vi "GetBusClass.vi"(8 "ErrorArray In":errorcluster[](array[cluster]), 9 "arg":string, 10 "BusNumber":u8) -> (0 "ErrorArray Out":errorcluster[](array[cluster]), 3 "Framework.lvlib:Bus.lvclass":refnum<class "Bus.lvclass">)   [LabVIEW 2017, in "Bus_class.lvlib" / "Bus.lvclass"]
uses:
  Bus.lvclass
  <vilib>/Utility/error.llb/Error Cluster From Error Code.vi
  <vilib>/ErrorRing/Error Ring.xnode
  <userlib>/NIST/NISTErrorLib/NISTErrorLib.lvlib
  Framework.lvlib
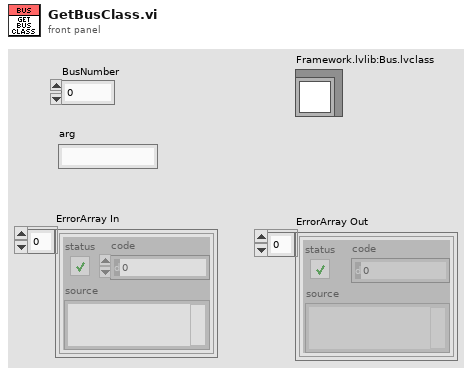
[diagram p1: front panel]
types:
  T1 = typedef "Framework.lvlib/clFrameworkData.ctl" = cluster{"EvtINIFilePaths":path[], "BusClassInstances":refnum<class "Bus.lvclass">[], "PmuImpairINIFilePaths":path[], "FlagImpairINIFilePaths":path[], "NetImpairINIFilePaths":path[], "OutputToFileINIFilePaths":path[], "AppINIFilePaths":path[], "AppModuleID":i32, "OutputToFileID":i32}
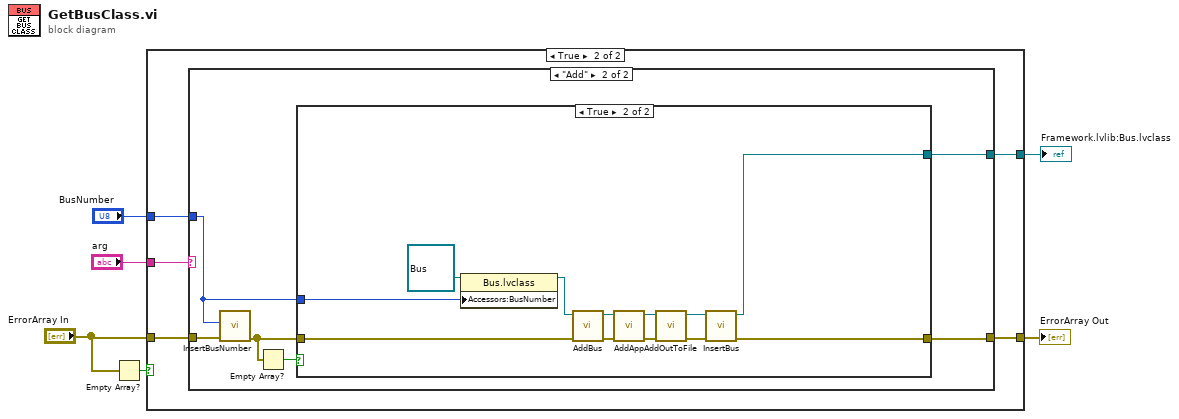
[diagram p0: block diagram]
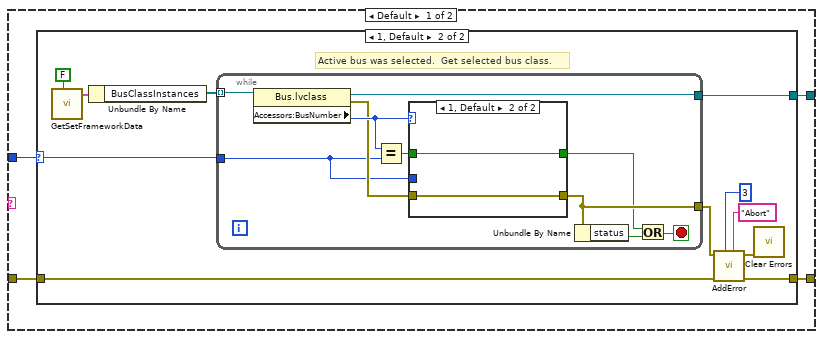
[diagram p3: hidden frame]
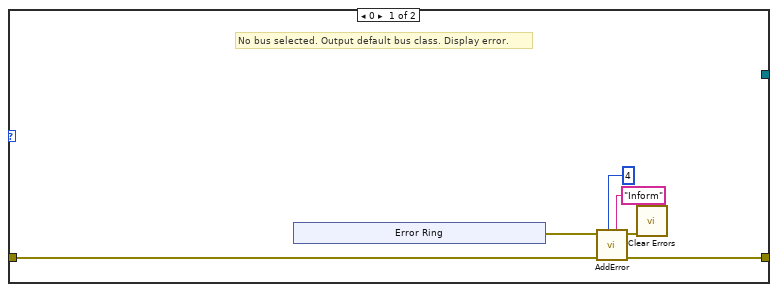
[diagram p4: hidden frame]
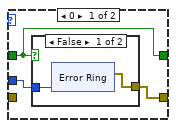
[diagram p5: hidden frame]
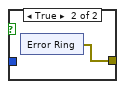
[diagram p6: hidden frame]
diagram:
  n1 = Empty Array?(array="ErrorArray In") -> (empty?=w2:bool)
  n2 = case shown="True" w2 {
    tunnel: "ErrorArray In" -> [w7 w11]
    tunnel: [w7 w12] -> w6
    tunnel: [_ w10] -> w5
    tunnel: "BusNumber" -> [_ w9]
    tunnel: "arg" -> [_ w8]
    frame False {
      # "External error.  Error array holds at least one error."
    }
    frame True {
      n3 = case shown="\"Add\"" w8 {
        tunnel: [w16 w70] -> w12
        tunnel: w11 -> [w15 w74]
        tunnel: [w14 w69] -> w10
        tunnel: w9 -> [w13 w71]
        frame Default {
          n4 = case shown="1, Default" w13 {
            selector: w13 -> [_ w32]
            tunnel: [w18 w38] -> w16
            tunnel: w15 -> [w19 w29]
            tunnel: [_ w31] -> w14
            frame 0 {
              # "No bus selected. Output default bus class. Display error."
              n5 = xnode "Error Ring"() -> ("error out"=w17:errorcluster)
              n6 = call <userlib>:"AddError.vi"("Severity"="Inform" ("String"), "Priority"=u8 4, "ErrorArray"=w19, "error in (no error)"=w17) -> ("ErrorArray"=w18:errorcluster[], "error out"=w22:errorcluster)  [unwired: 6 in]
              n7 = call <vilib>:"Clear Errors.vi"("error in (no error)"=w22) -> ()  [unwired: 5 in, 2 out]
            }
            frame 1, Default {
              # "Active bus was selected.  Get selected bus class."
              n8 = call "GetSetFrameworkData.vi"("Set (F)"=FALSE ("Set/Get")) -> ("clFrameworkData Out"=w33:T1)  [unwired: 10 in]
              n9 = Unbundle By Name(w33) -> ("BusClassInstances"=w30:refnum<class "Bus.lvclass">[])
              n10 = while {
                tunnel: w32 -> [w41]
                tunnel: [w48] -> w31
                tunnel: w30 -> [w47] mode=indexing
                tunnel: [w42] -> w28
                stop <- w45 stop-if-true
                n11 = property class="Bus.lvclass"(reference=w47) -> (reference out=w48:refnum<class "Bus.lvclass">, error out=w43:errorcluster, "Accessors:BusNumber"=w44:u8)  [unwired: 1 in]
                n12 = Equal?(x=w44, y=w41) -> (x = y?=w40:bool)
                n13 = case shown="1, Default" w44 {
                  tunnel: [w50 w68] -> w42
                  tunnel: w43 -> [_ w68]
                  tunnel: w41 -> [w49 _]
                  tunnel: w40 -> [w51 w67]
                  tunnel: [w51 w67] -> w39
                  frame 0 {
                    n14 = case shown="False" w51 {
                      tunnel: [w53 w61] -> w50
                      tunnel: w49 -> [w52 _]
                      frame False {
                        n15 = xnode "Error Ring"("parameter 0"=w52) -> ("error out"=w53:errorcluster)
                      }
                      frame True {
                        n16 = xnode "Error Ring"() -> ("error out"=w61:errorcluster)
                      }
                    }
                  }
                  frame 1, Default {
                  }
                }
                n17 = Unbundle By Name(w42) -> ("status"=w46:bool)
                n18 = Or(x=w39, y=w46) -> (x .or. y?=w45:bool)
              }
              n19 = call <userlib>:"AddError.vi"("Severity"="Abort" ("String"), "Priority"=u8 3, "ErrorArray"=w29, "error in (no error)"=w28) -> ("ErrorArray"=w38:errorcluster[], "error out"=w37:errorcluster)  [unwired: 6 in]
              n20 = call <vilib>:"Clear Errors.vi"("error in (no error)"=w37) -> ()  [unwired: 5 in, 2 out]
            }
          }
        }
        frame "Add" {
          n21 = call "InsertBusNumber.vi"("ErrorArray In"=w74, "BusNumber"=w71) -> ("ErrorArray Out"=w73:errorcluster[])  [unwired: 9 in]
          n22 = Empty Array?(array=w73) -> (empty?=w72:bool)
          n23 = case shown="True" w72 {
            tunnel: w73 -> [w75 w85]
            tunnel: w71 -> [_ w86]
            tunnel: [w75 w77] -> w70
            tunnel: [_ w76] -> w69
            frame False {
            }
            frame True {
              n24 = property class="Bus.lvclass"(reference=refnum<class "Bus.lvclass"> refnum ("Bus_class.lvlib:Bus.lvclass"), "Accessors:BusNumber"=w86) -> (reference out=w84:refnum<class "Bus.lvclass">)  [unwired: 1 in, 1 out]
              n25 = call "AddBus.vi"("ErrorArray In"=w85, "BusClass In"=w84) -> ("ErrorArray Out"=w83:errorcluster[], "BusClass Out"=w82:refnum<class "Bus.lvclass">)  [unwired: 7 in, 1 out]
              n26 = call "AddApp.vi"("ErrorArray In"=w83, "BusClass In"=w82) -> ("ErrorArray Out"=w81:errorcluster[], "BusClass Out"=w80:refnum<class "Bus.lvclass">)  [unwired: 7 in, 1 out]
              n27 = call "AddOutToFile.vi"("ErrorArray In"=w81, "BusClass In"=w80) -> ("ErrorArray Out"=w79:errorcluster[], "BusClass Out"=w78:refnum<class "Bus.lvclass">)  [unwired: 7 in, 1 out]
              n28 = call "InsertBus.vi"("ErrorArray In"=w79, "BusClass In"=w78) -> ("ErrorArray Out"=w77:errorcluster[], "BusClass Out"=w76:refnum<class "Bus.lvclass">)  [unwired: 8 in]
            }
          }
        }
      }
    }
  }
  "Framework.lvlib:Bus.lvclass" <- w5
  "ErrorArray Out" <- w6
